vi "lvRunVi.vi"() -> (0 "error out":errorcluster)   [LabVIEW 2014, in "lvcommonbuild.lvlib"]
uses:
  lvcommonbuild.lvlib
  <vilib>/Wiresmith Technology/LabVIEW CLI/CLI Class/CLI.lvclass
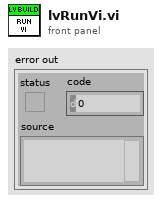
[diagram p1: front panel]
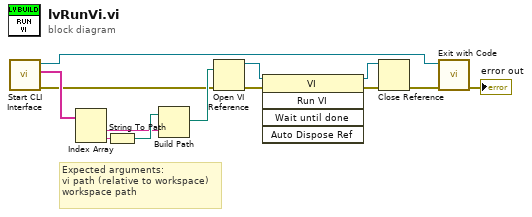
[diagram p0: block diagram]
diagram:
  # "Expected arguments:\nvi path (relative to workspace)\nworkspace path"
  n1 = call <vilib>:"Start CLI Interface.vi"() -> ("error out"=w4:errorcluster, "Custom Parameters"=w13:string[], "CLI out"=w3:refnum<class "CLI.lvclass">)  [unwired: 9 in]
  n2 = Index Array(array=w13) -> (element #1=w2:string, element #2=w10:string)  [unwired: 2 in]
  n3 = String To Path(string=w10) -> (path=w11:path)
  n4 = Build Path(base path=w11, name or relative path=w2) -> (appended path=w9:path)
  n5 = Open VI Reference(vi path=w9, error in (no error)=w4) -> (vi reference=w7:refnum<vi>, error out=w8:errorcluster)  [unwired: 4 in]
  n6 = invoke class="VI" method="Run VI"(reference=w7, error in=w8) -> (reference out=w5:refnum<vi>, error out=w6:errorcluster)  [unwired: 3 in, 3 out]
  n7 = Close Reference(reference=w5, error in (no error)=w6) -> (error out=w1:errorcluster)
  n8 = call <vilib>:"Exit with Code.vi"("error in (no error)"=w1, "CLI in"=w3) -> ("error out"=→"error out":errorcluster)  [unwired: 9 in]
